vi "LinkTest.vi"() -> (0 "error out":errorcluster, 2 "pass":bool)   [LabVIEW 2025, in "NISE_CEF_Tests.lvlib"]
uses:
  NISE_CEF_Tests.lvlib
  Trunk/ProjectTemplates/Source/Configuration Editor Framework/Classes/cRIO/cRIO.lvclass
  Trunk/ProjectTemplates/Source/Configuration Editor Framework/Classes/cRIO Repo/cRIORepo.lvclass
  Trunk/Configuration Framework/Node/Summary.ctl
  Controls/IDs.ctl
panel:
  out "Ids":T1
  out "summary 2":T2[](array[typedef])
  in  "number of nodes":i32
  out "summary":T2[](array[typedef])
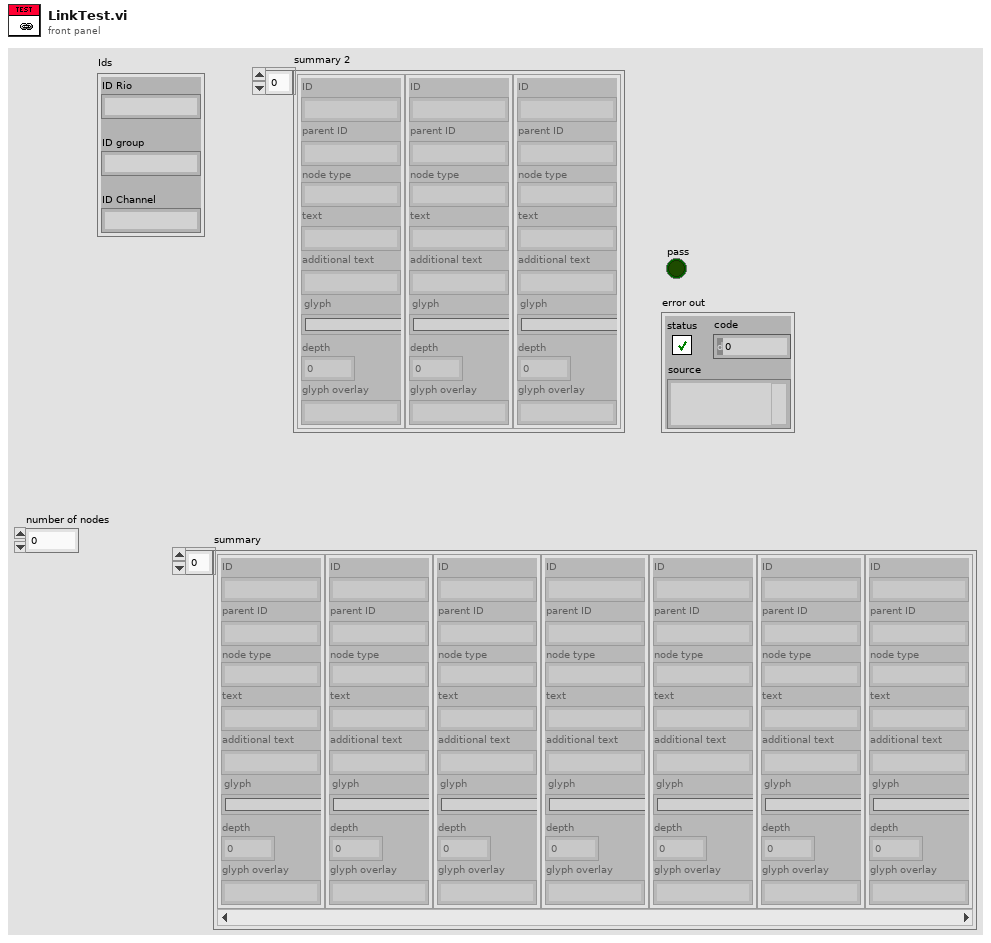
[diagram p1: front panel]
types:
  T1 = typedef "NISE_CEF_Tests.lvlib/IDs.ctl" = cluster{"ID Channel":string, "ID Rio":string, "ID group":string}
  T2 = typedef "NISE_CEF_Node.lvclass/Summary.ctl" = cluster{"ID":string, "parent ID":string, "node type":string, "text":string, "additional text":string, "glyph":string, "depth":i32, "glyph overlay":string}
  T3 = typedef "NISE_CEF_Node.lvclass/NodeRef.ctl" = refnum<data-value>
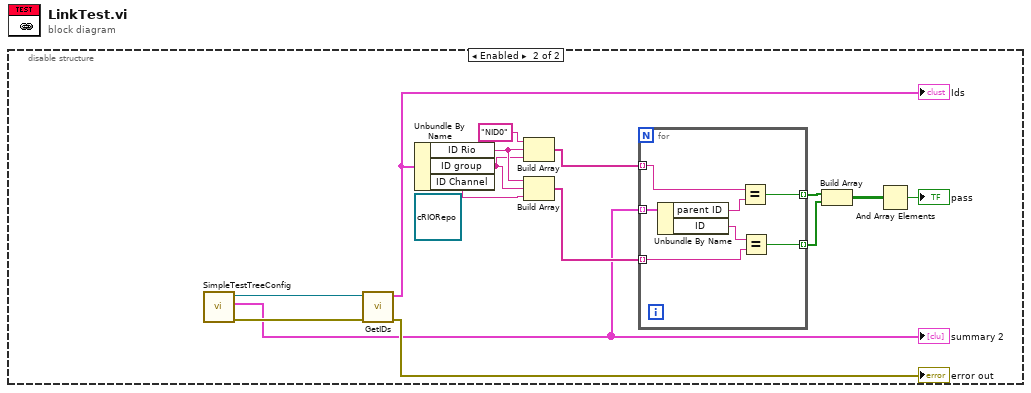
[diagram p0: block diagram]
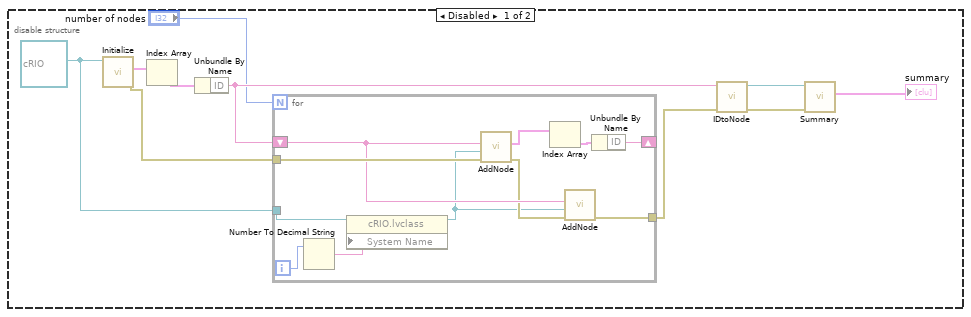
[diagram p2: hidden frame]
diagram:
  n1 = disable-structure shown="Enabled" {
    frame Disabled {
      w1 = refnum<class "cRIO.lvclass"> refnum ("cRIO.lvclass")
      n2 = call-dynamic "Initialize.vi"("cRIO in"=w1) -> ("error out"=w7:errorcluster, "summary"=w10:T2[])  [unwired: 8 in, 1 out]
      n3 = Index Array(array=w10) -> (element=w9:T2)  [unwired: 1 in]
      n4 = Unbundle By Name(w9) -> ("ID"=w8:string)
      n5 = for {
        N: "number of nodes" -> [_]
        tunnel: w1 -> [w14]
        shift-right: [w19] -> _
        shift-left: w8 -> [w17]
        tunnel: w7 -> [w18]
        tunnel: [w15] -> w3
        i -> [w13]
        n6 = Number To Decimal String(number=w13) -> (decimal integer string=w12:string)  [unwired: 1 in]
        n7 = property class="cRIO.lvclass"(reference=w14, "System Name"=w12) -> (reference out=w11:refnum<class "cRIO.lvclass">)  [unwired: 1 in, 1 out]
        n8 = call "AddNode.vi"("error in"=w18, "node in"=w11, "parent node ID"=w17) -> ("error out"=w16:errorcluster, "summary"=w20:T2[])  [unwired: 7 in]
        n9 = Index Array(array=w20) -> (element=w21:T2)  [unwired: 1 in]
        n10 = call "AddNode.vi"("error in"=w16, "node in"=w11, "parent node ID"=w17) -> ("error out"=w15:errorcluster)  [unwired: 7 in, 1 out]
        n11 = Unbundle By Name(w21) -> ("ID"=w19:string)
      }
      n12 = call "IDtoNode.vi"("error in"=w3, "ID"=w8) -> ("error out"=w2:errorcluster, "node ref"=w4:T3)  [unwired: 7 in, 1 out]
      n13 = call "Summary.vi"("error in"=w2, "node self ref"=w4) -> ("summary"=→"summary":T2[])  [unwired: 8 in, 1 out]
    }
    frame Enabled {
      (unwired) refnum<class "cRIORepo.lvclass"> refnum ("cRIORepo.lvclass")
      n14 = call "SimpleTestTreeConfig.vi"() -> ("error out"=w36:errorcluster, "summary"=w22:T2[], "Data Value Reference out"=w34:T3)  [unwired: 9 in]
      "summary 2" <- w22
      n15 = call "GetIDs.vi"("error in"=w36, "data value reference in"=w34) -> ("error out"=→"error out":errorcluster, "IDs"=w29:T1)  [unwired: 6 in, 2 out]
      "Ids" <- w29
      n16 = Unbundle By Name(w29) -> ("ID Rio"=w28:string, "ID group"=w27:string, "ID Channel"=w26:string)
      n17 = Build Array("NID0" ("parent ID"), w28, w27) -> (w32:string[])
      n18 = Build Array(w28, w27, w26) -> (w25:string[])
      n19 = for {
        tunnel: w22 -> [w43] mode=indexing
        tunnel: w32 -> [w41] mode=indexing
        tunnel: [w42] -> w31 mode=indexing
        tunnel: w25 -> [w38] mode=indexing
        tunnel: [w37] -> w23 mode=indexing
        n20 = Unbundle By Name(w43) -> ("parent ID"=w40:string, "ID"=w39:string)
        n21 = Equal?(x=w41, y=w40) -> (x = y?=w42:bool)
        n22 = Equal?(x=w39, y=w38) -> (x = y?=w37:bool)
      }
      n23 = Build Array(w31, w23) -> (w24:bool[][])
      n24 = And Array Elements(Boolean array=w24) -> (logical AND=→"pass":bool)
    }
  }
